vi "Connection Manager (general).vi"(7 "Path":path, 8 "color":u32(colorbox)=16762479, 9 "Custom Inputs":string[](array[string]), 10 "Properties In":variant, 11 "Custom Outputs":string[](array[string])) -> (2 "Properties Out":variant)   [LabVIEW 2020]
uses:
  Type Defs/General PXISlot XControl/PXISlotGP.xctl
  Utility VIs/Buttons/KCheckmarkBoolean 2.ctl
  Utility VIs/Controls/KPropertyTable/KPropertyTable.xctl
  Utility VIs/Controls/KBackground Gradient/KBackground Gradient.xctl
panel:
  in  "Properties":T1[](xcontrol)
  in  "Hide unused":T3
  in  "Exit":bool
  in  "Save":bool
  in  "KBackground":dbl(xcontrol)
  in  "Slot3":cluster{"Outputs":string[], "Inputs":string[]}(xcontrol) caption="Slot 3"
  in  "Slot2":cluster{"Outputs":string[], "Inputs":string[]}(xcontrol) caption="Slot 2"
  in  "Slot9":cluster{"Outputs":string[], "Inputs":string[]}(xcontrol) caption="Slot 3"
  in  "Slot8":cluster{"Outputs":string[], "Inputs":string[]}(xcontrol) caption="Slot 8"
  in  "Slot7":cluster{"Outputs":string[], "Inputs":string[]}(xcontrol) caption="Slot 7"
  in  "Slot6":cluster{"Outputs":string[], "Inputs":string[]}(xcontrol) caption="Slot 6"
  in  "Slot5":cluster{"Outputs":string[], "Inputs":string[]}(xcontrol) caption="Slot 5"
  in  "Slot4":cluster{"Outputs":string[], "Inputs":string[]}(xcontrol) caption="Slot 2"
  # "Inputs"
  # "Outputs"
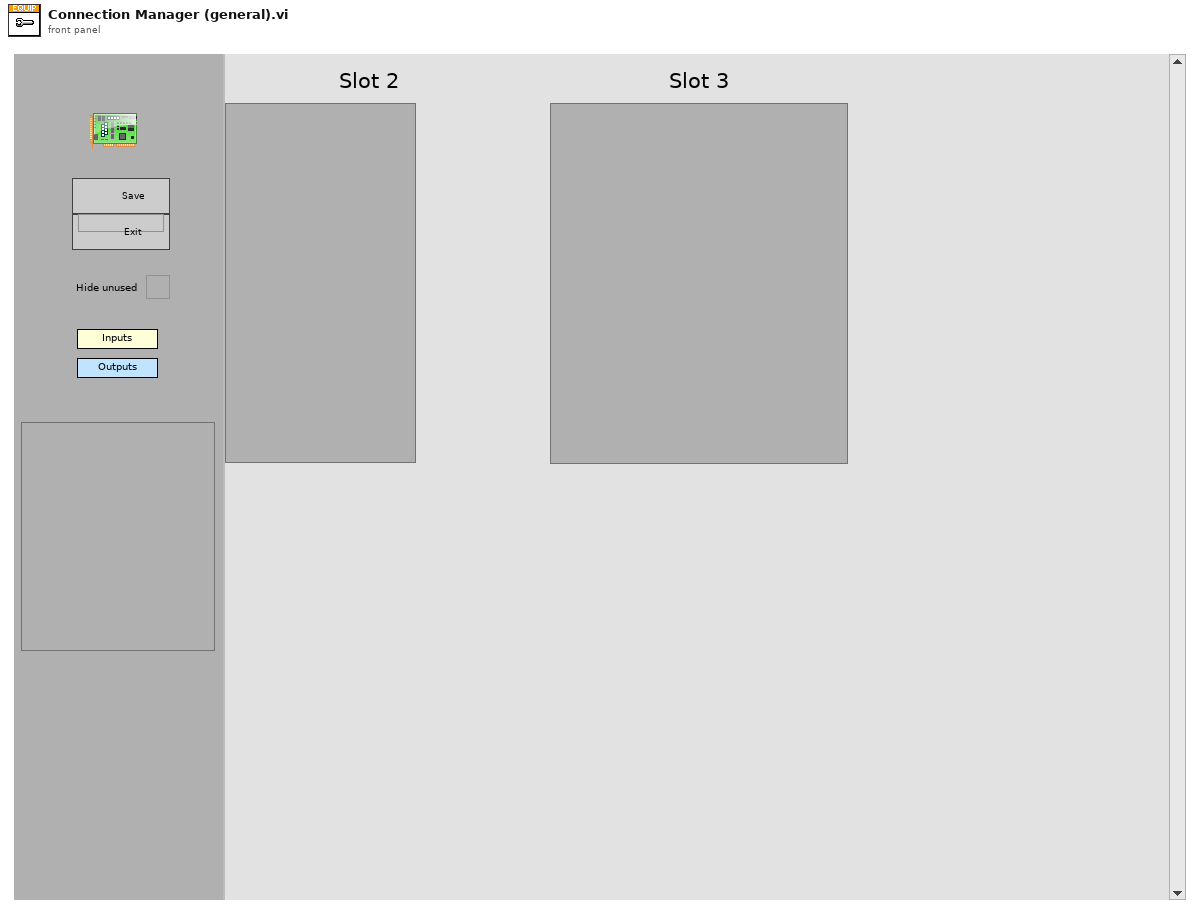
[diagram p1: front panel]
types:
  T1 = typedef "KPropertyTable.xctl/RowData.ctl" = cluster{"Name":string, "Type":T2, "Category":string, "Strings":string[], "Value":string}
  T2 = typedef "KPropertyTable.xctl/DataType.ctl" = enum16{"String", "Enum", "Int", "Double", "Boolean", "Ring", "Formula"}
  T3 = typedef "KCheckmarkBoolean 2.ctl" = bool
  T4 = typedef "PXI-Device Spec.ctl" = cluster{"Slot":i32, "ProductType":string, "NumAO":i32, "NumAI":i32, "Device Name":string}
  T5 = cluster{"AO Endpoints":string[], "AI Endpoints":string[]}[]
  T6 = cluster{"Custom Inputs":string[], "Custom Outputs":string[]}
  T7 = typedef "Connector Type.ctl" = enum16{"None", "PXI-4461", "BNC-2110", "BNC-2090", "PXIe-4463", "PXIe-4464"}
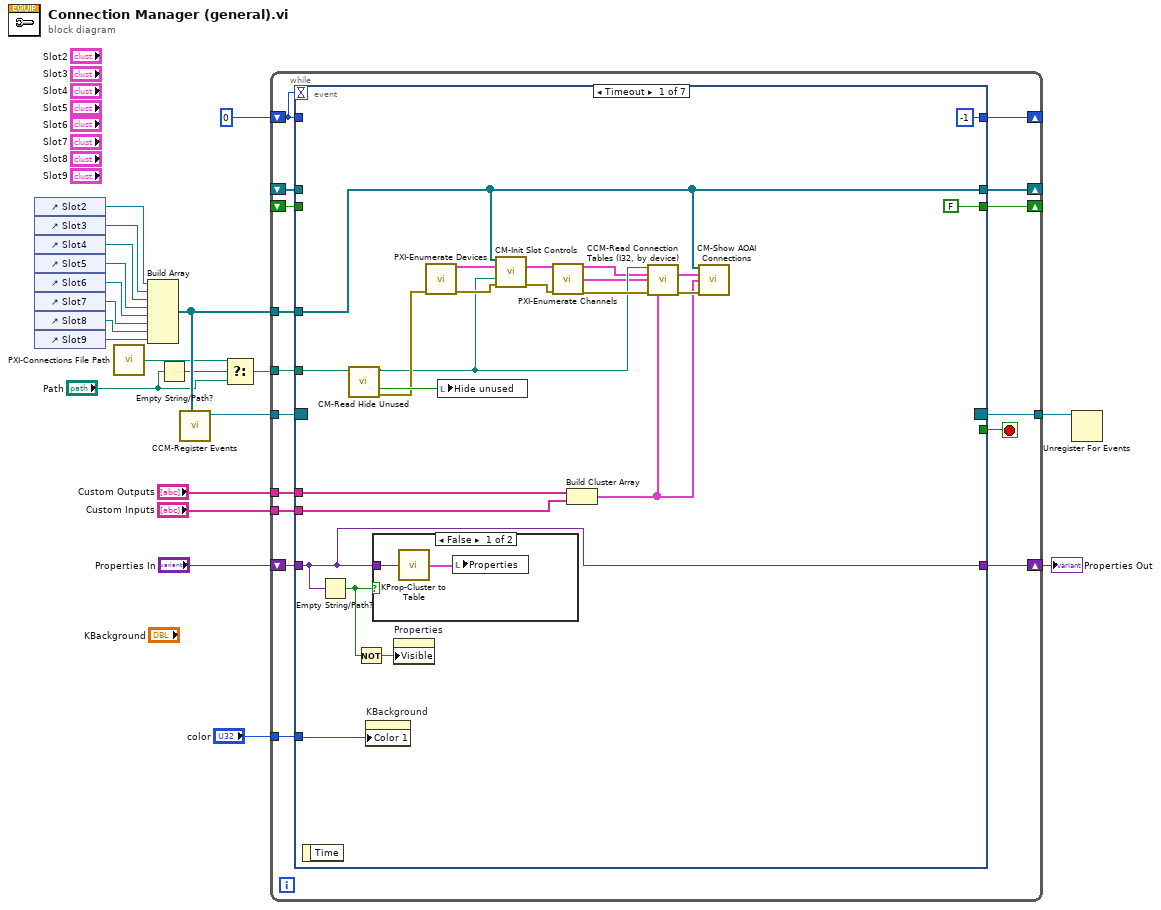
[diagram p0: block diagram]
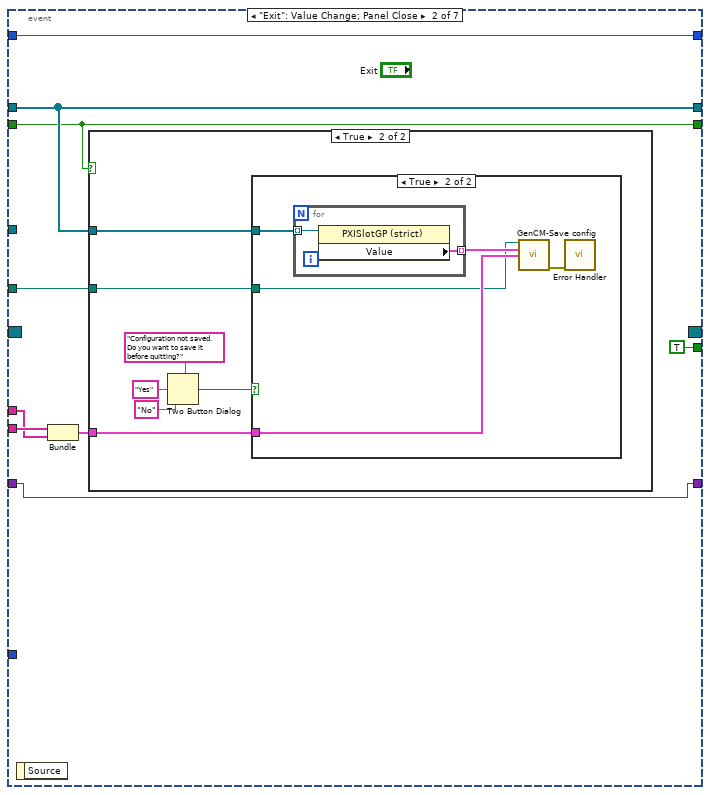
[diagram p3: hidden frame]
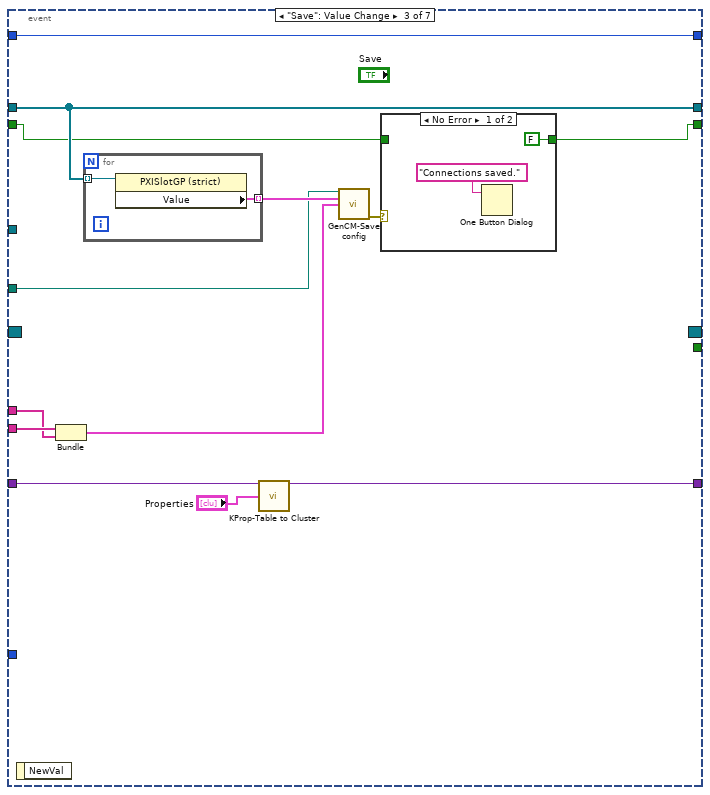
[diagram p6: hidden frame]
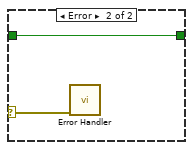
[diagram p7: hidden frame]
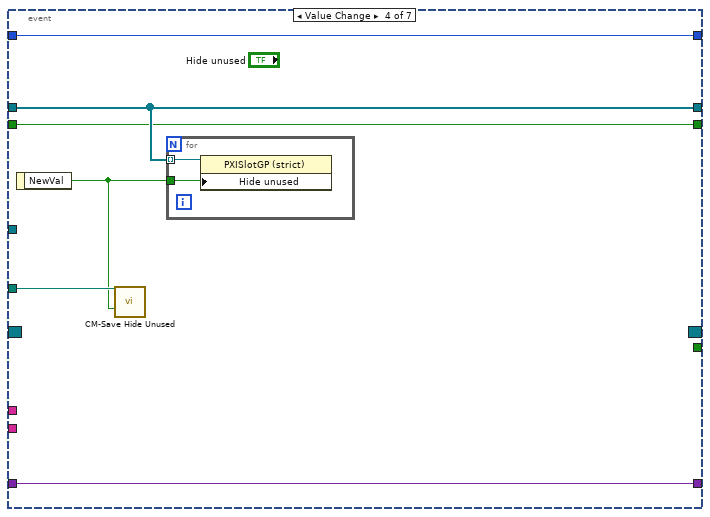
[diagram p8: hidden frame]
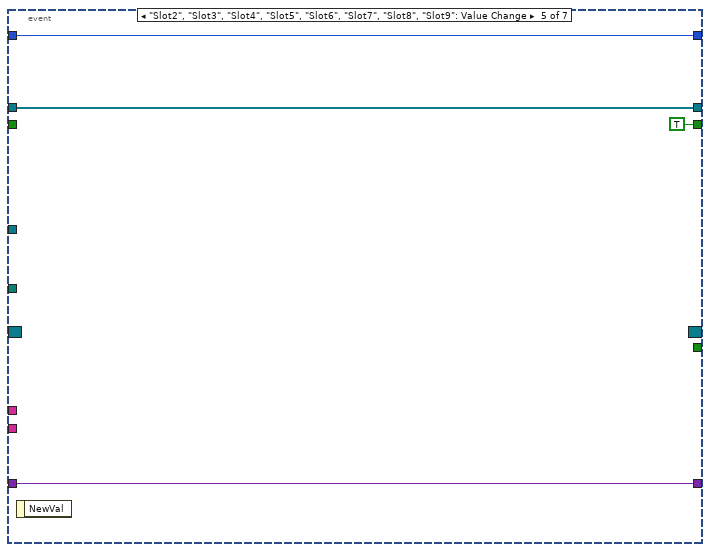
[diagram p9: hidden frame]
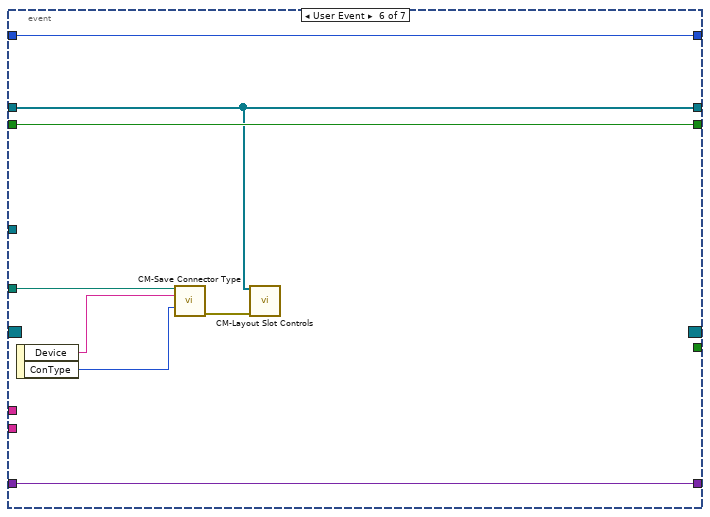
[diagram p10: hidden frame]
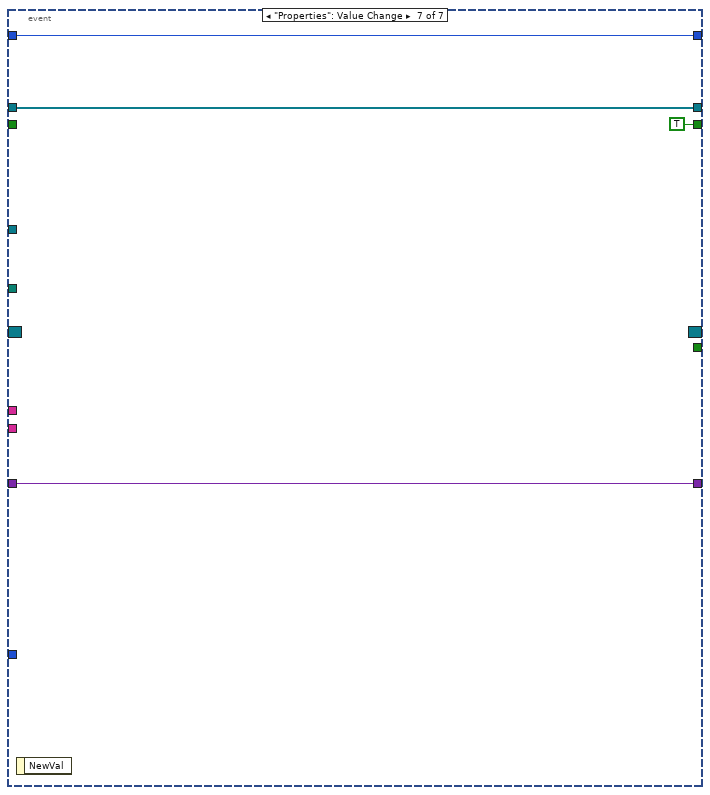
[diagram p11: hidden frame]
diagram:
  n1 = control-ref of="Slot2"() -> (w14:refnum<vi>)
  n2 = control-ref of="Slot3"() -> (w13:refnum<vi>)
  n3 = control-ref of="Slot4"() -> (w12:refnum<vi>)
  n4 = control-ref of="Slot5"() -> (w11:refnum<vi>)
  n5 = control-ref of="Slot6"() -> (w15:refnum<vi>)
  n6 = control-ref of="Slot7"() -> (w16:refnum<vi>)
  n7 = control-ref of="Slot8"() -> (w17:refnum<vi>)
  n8 = control-ref of="Slot9"() -> (w18:refnum<vi>)
  n9 = call "PXI-Connections File Path.vi"() -> ("Path"=w6:path)  [unwired: 1 in]
  n10 = Build Array(w14, w13, w12, w11, w15, w16, w17, w18) -> (w10:refnum<vi>[])
  n11 = Empty String/Path?(string/path="Path") -> (empty?=w5:bool)
  n12 = call "CCM-Register Events.vi"("Conn Refs"=w10) -> ("Event Registration Refnum"=w9:refnum<event-registration>)  [unwired: 8 in, 2 out]
  n13 = Select(t=w6, s=w5, f="Path") -> (s? t:f=w7:path)
  n14 = while {
    shift-right: [w36] -> _
    shift-left: 0 -> [w27]
    shift-right: [w34] -> _
    shift-left: _ -> [w35]
    tunnel: "Custom Outputs" -> [w33]
    tunnel: "Custom Inputs" -> [w32]
    tunnel: w10 -> [w31]
    tunnel: w7 -> [w30]
    shift-right: [w29] -> _
    shift-left: _ -> [w28]
    tunnel: w9 -> [w26]
    tunnel: [w25] -> w8
    tunnel: "color" -> [w24]
    shift-right: [w22] -> w1
    shift-left: "Properties In" -> [w23]
    stop <- w37 stop-if-true
    n15 = event shown="[0] Timeout" {
      selector: w26 -> [_ _ _ _ _ _ _]
      dyn-events: [_ _ _ _ _ _ _] -> w25
      timeout: w27 -> [_ _ _ _ _ _ _]
      tunnel: [_ TRUE _ _ _ _ _] -> w37
      tunnel: [-1 w64 w92 w106 w114 w124 w128] -> w36
      tunnel: [w54 w70 w98 w110 w116 w118 w127] -> w34
      tunnel: w35 -> [_ w70 w98 w110 w116 w118 w127]
      tunnel: w33 -> [w52 w67 w94 _ _ _ _]
      tunnel: w32 -> [w51 w68 w95 _ _ _ _]
      tunnel: w31 -> [w54 _ _ _ _ _ _]
      tunnel: w30 -> [w49 w65 w91 w109 _ w122 _]
      tunnel: [FALSE w66 w89 w107 TRUE w123 TRUE] -> w29
      tunnel: w28 -> [_ w66 w90 w107 _ w123 _]
      tunnel: w27 -> [_ w64 w92 w106 w114 w124 w128]
      tunnel: w24 -> [w38 _ _ _ _ _ _]
      tunnel: w23 -> [w39 w63 w87 w105 w113 w117 w126]
      tunnel: [w39 w63 w86 w105 w113 w117 w126] -> w22
      event Timeout {
        n16 = event-data() -> ()  [unwired: 1 in, 1 out]
        n17 = Empty String/Path?(string/path=w39) -> (empty?=w40:bool)
        n18 = call "CM-Read Hide Unused.vi"("configuration file path"=w49) -> ("file path"=w47:path, "Hide unused"=w50:bool, "error out"=w48:errorcluster)  [unwired: 12 in]
        n19 = Not(x=w40) -> (.not. x?=w41:bool)
        n20 = property on="KBackground" class="KBackground Gradient (strict)"("Color 1"=w38) -> ()  [unwired: 2 in, 2 out]
        n21 = case shown="False" w40 {
          tunnel: w39 -> [w62 _]
          frame False {
            n22 = call "KProp-Cluster to Table.vi"("Anything"=w62) -> ("Rows"=w61:T1[])  [unwired: 13 in, 1 out]
            n23 = local write "Properties"(w61) -> ()
          }
          frame True {
          }
        }
        n24 = property on="Properties" class="KPropertyTable (strict)"("Visible"=w41) -> ()  [unwired: 2 in, 2 out]
        n25 = call "PXI-Enumerate Devices.vi"("error in (no error)"=w48) -> ("Devices"=w59:T4[], "error out"=w55:errorcluster)  [unwired: 13 in]
        n26 = local write "Hide unused"(w50) -> ()
        n27 = call "CM-Init Slot Controls.vi"("slot ctl refs"=w54, "Devices"=w59, "config file"=w47, "error in (no error)"=w55) -> ("Devices thru"=w58:T4[], "error out"=w56:errorcluster)  [unwired: 9 in, 1 out]
        n28 = call "PXI-Enumerate Channels.vi"("Devices"=w58, "error in (no error)"=w56) -> ("Channels By Device"=w45:cluster{"Out":string[], "In":string[]}[], "Channels (1D)"=w44:cluster{"Out":string[], "In":string[]}, "error out"=w57:errorcluster)  [unwired: 11 in]
        n29 = Build Cluster Array(w52, w51) -> (w43:cluster{"Custom Inputs":string[]}[])
        n30 = call "CCM-Read Connection Tables (I32, by device).vi"("Path In"=w47, "Channels By Device"=w45, "Channels (1D)"=w44, "error in (no error)"=w57, "Endpoints"=w43) -> ("Tables By Device"=w46:T5, "error out"=w53:errorcluster)  [unwired: 8 in, 1 out]
        n31 = call "CM-Show AOAI Connections.vi"("slot ctl refs"=w54, "Tables By Device"=w46, "Endpoints"=w43, "error in (no error)"=w53) -> ()  [unwired: 10 in, 2 out]
      }
      event "Exit": Value Change; Panel Close {
        n32 = event-data() -> ()  [unwired: 1 in, 1 out]
        n33 = Bundle("Custom Inputs"=w68, "Custom Outputs"=w67) -> (w69:T6)  [unwired: 1 in]
        n34 = case shown="True" w66 {
          tunnel: w70 -> [_ w74]
          tunnel: w69 -> [_ w73]
          tunnel: w65 -> [_ w72]
          frame False {
          }
          frame True {
            n35 = Two Button Dialog(message="Configuration not saved. Do you want to save it before quitting?", 1:"No" ("F button name (\"Cancel\")"), 2:"Yes" ("T button name (\"OK\")")) -> (T button?=w75:bool)
            n36 = case shown="True" w75 {
              tunnel: w74 -> [_ w82]
              tunnel: w73 -> [_ w80]
              tunnel: w72 -> [_ w79]
              frame False {
              }
              frame True {
                n37 = for {
                  tunnel: w82 -> [w85] mode=indexing
                  tunnel: [w84] -> w81 mode=indexing
                  n38 = property class="PXISlotGP (strict)"(reference=w85) -> ("Value"=w84:cluster{"Outputs":string[], "Inputs":string[]})  [unwired: 1 in, 2 out]
                }
                n39 = call "GenCM-Save config.vi"("configuration file path"=w79, "Analog Connections"=w81, "Endpoints"=w80) -> ("error out"=w83:errorcluster)  [unwired: 12 in]
                n40 = call "Error Handler.vi"("error in (no error)"=w83) -> ()  [unwired: 13 in, 2 out]
              }
            }
          }
        }
      }
      event "Save": Value Change {
        n41 = event-data() -> ()  [unwired: 1 in, 1 out]
        n42 = Bundle("Custom Inputs"=w95, "Custom Outputs"=w94) -> (w96:T6)  [unwired: 1 in]
        n43 = for {
          tunnel: w98 -> [w104] mode=indexing
          tunnel: [w103] -> w97 mode=indexing
          n44 = property class="PXISlotGP (strict)"(reference=w104) -> ("Value"=w103:cluster{"Outputs":string[], "Inputs":string[]})  [unwired: 1 in, 2 out]
        }
        n45 = call "KProp-Table to Cluster.vi"("Anything"=w87, "Rows"="Properties") -> ("variant"=w86:variant)  [unwired: 12 in, 1 out]
        n46 = call "GenCM-Save config.vi"("configuration file path"=w91, "Analog Connections"=w97, "Endpoints"=w96) -> ("error out"=w93:errorcluster)  [unwired: 12 in]
        n47 = case shown="No Error" w93 {
          selector: w93 -> [_ w102]
          tunnel: w90 -> [_ w101]
          tunnel: [FALSE w101] -> w89
          frame No Error {
            n48 = One Button Dialog(message="Connections saved.") -> ()  [unwired: 1 in, 1 out]
          }
          frame Error {
            n49 = call "Error Handler.vi"("error in (no error)"=w102) -> ()  [unwired: 13 in, 2 out]
          }
        }
      }
      event Value Change {
        n50 = event-data() -> ("NewVal"=w108:T3)  [unwired: 1 in]
        n51 = call "CM-Save Hide Unused.vi"("configuration file path"=w109, "Hide unused"=w108) -> ()  [unwired: 12 in, 2 out]
        n52 = for {
          tunnel: w110 -> [w112] mode=indexing
          tunnel: w108 -> [w111]
          n53 = property class="PXISlotGP (strict)"(reference=w112, "Hide unused"=w111) -> ()  [unwired: 1 in, 2 out]
        }
      }
      event "Slot2", "Slot3", "Slot4", "Slot5", "Slot6", "Slot7", "Slot8", "Slot9": Value Change {
        n54 = event-data() -> ()  [unwired: 1 in, 1 out]
      }
      event User Event {
        n55 = event-data() -> ("Device"=w121:string, "ConType"=w120:T7)  [unwired: 1 in]
        n56 = call "CM-Save Connector Type.vi"("configuration file path"=w122, "Device"=w121, "ConType"=w120) -> ("error out"=w119:errorcluster)  [unwired: 11 in, 1 out]
        n57 = call "CM-Layout Slot Controls.vi"("SlotRefs"=w118, "error in (no error)"=w119) -> ()  [unwired: 13 in, 1 out]
      }
      event "Properties": Value Change {
        n58 = event-data() -> ()  [unwired: 1 in, 1 out]
      }
    }
  }
  "Properties Out" <- w1
  n59 = Unregister For Events(event registration refnum=w8) -> ()  [unwired: 1 in, 1 out]
